vi "VI LogKonfig.vi"() -> ()   [LabVIEW 2020, in "LogKonfig.lvlib"]
uses:
  Seiten/Log Konfig/LogKonfig.lvlib
  Visualisierungs Elemente/String - Eingabefeld.ctl
  Visualisierungs Elemente/Pfad-Eingabefeld.ctl
  Visualisierungs Elemente/Button.ctl
  Visualisierungs Elemente/Auswahlfeld.ctl
  Visualisierungs Elemente/Zahlen-Eingabefeld.ctl
  Linearisierung V2/AktivButton.ctl
  Seiten/FT-IR/FGV FT-IR Aktionen.ctl
  Seiten/Log Konfig/Aktionen Logdatei erstellen.ctl
  Seiten/Log Konfig/Aktionen Trigger.ctl
  Seiten/FT-IR/FGV FT-IR Gasliste Aktionen.ctl
  Seiten/Log Konfig/Aktion LabBaseIndex.ctl
  Seiten/Log Konfig/Log Sequence FGV Aktion.ctl
  Passwortverwaltung/FGV Passwort Aktion.ctl
  SysLog/SysLog Interface.ctl
  Seiten/Log Konfig/Element Triggerereignisse.ctl
  Seiten/Log Konfig/Auswahlfeld aktiviert-deaktiviert.ctl
  Seiten/FT-IR/FT-IR.lvlib
  Seiten/FT-IR/TOOLweb Interface Library/TOOLweb Interface.lvlib
  Passwortverwaltung/Passwort.lvlib
  Allgemein/allgemeine Sub-VIs.lvlib
  Messdaten/Messdaten.lvlib
  SysLog/SysLog.lvlib
  Linearisierung V2/Linearisierung v2.lvlib
panel:
  in  "Registerkartenelement":T1(tab)
  out "Index Nr.":u32 caption="SPEC#:"
  in  "Index Nr. Start:":u32 caption="SPEC#:"
  in  "Logdatei erstellen":u16(ring) items=["Deaktiviert", "Aktiviert"]
  in  "Name":T2
  in  "Pfad LogDatei":T3
  in  "Trigger verwenden":u16(ring) items=["Deaktiviert", "Aktiviert"]
  in  "Puffergröße":T4 format="%#_5g"
  in  "Triggerereignis":T5
  in  "Messwert":T6 items=["---"]
  in  "kl./gr.":T6 items=["kleiner", "größer"]
  in  "Wert":T4 format="%#_5g"
  in  "Spektrum Loggen":u16(ring) items=["Deaktiviert", "Aktiviert"]
  in  "Pfad Spektren":T3
  in  "(82) labBaseName":T2
  in  "max. Größe  in Byte":u32=31457280 caption="max. Größe in Byte" min=15000 format="%#.0f"
  in  "Original Liste":i32(listbox)
  in  "Übernehmen":T5
  in  "Konfigurierte Liste":i32(listbox)
  in  "Löschen":T5
  in  "Alle Löschen":T5
  in  "Alle Übernehmen":T5
  in  "Spektrum File Name":T7 caption="Spektrum Datei Name"
  # "Log Konfig"
  # "FT-IR Spectrum"
  # "Spektrum Loggen?"
  # "Pfad für Spektren:"
  # "Bezeichnung:"
  # "Logdatei Messdaten"
  # "Logdatei erstellen?"
  # "Pfad für Logdatei:"
  # "Messreihenbezeichnung:"
  # "Trigger Einstellungen"
  # "-- Taste [F11]"
  # "--24V Trigger-Input"
  # "Trigger verwenden?"
  # "Triggerereignisse:"
  # "-- AK-Befehl [STRG]"
  # "sec"
  # "Puffergröße:"
  # "(Der Pufferbereich wird vor dem Triggerereignis mitgeloggt)"
  # "-- Messwert"
  # "Konfiguration Kanalreihenfolge"
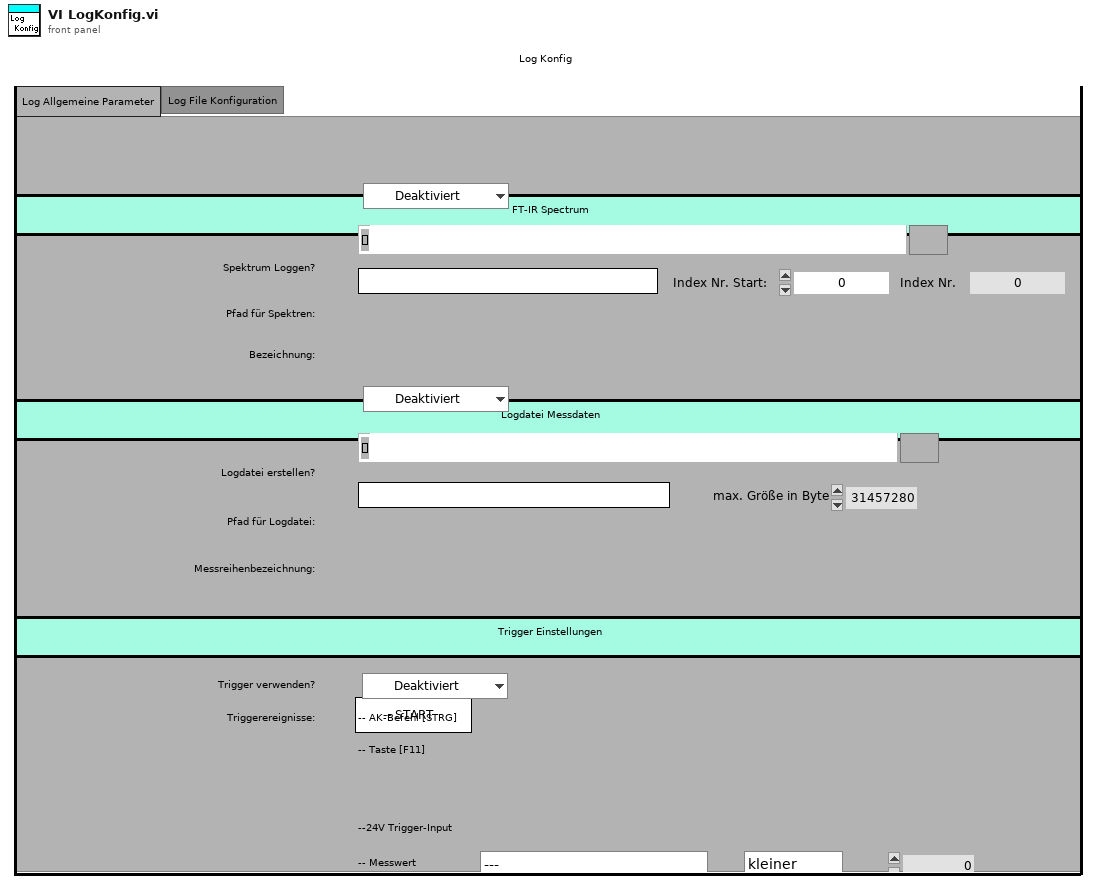
[diagram p1: front panel]
types:
  T1 = enum32{"Log General Parameter", "Log File Configuration"}
  T2 = typedef "String - Eingabefeld.ctl" = string
  T3 = typedef "Pfad-Eingabefeld.ctl" = path
  T4 = typedef "Zahlen-Eingabefeld.ctl" = sgl
  T5 = typedef "Button.ctl" = bool
  T6 = typedef "Auswahlfeld.ctl" = u16
  T7 = typedef "Linearisierung v2.lvlib/AktivButton.ctl" = bool
  T8 = typedef "LogKonfig.lvlib/Aktion LabBaseIndex.ctl" = enum16{"lesen", "schreiben"}
  T9 = typedef "FT-IR.lvlib/FGV FT-IR Gasliste Aktionen.ctl" = enum16{"lesen", "Gasliste FT-IR", "Gasliste ausgelesen", "laden", "speichern", "löschen"}
  T10 = typedef "LogKonfig.lvlib/Aktionen Trigger.ctl" = enum16{"lesen", "ALLE schreiben", "Trigger prüfen", "Trigger rücksetzen"}
  T11 = typedef "LogKonfig.lvlib/Aktionen Logdatei erstellen.ctl" = enum16{"lesen", "Logdatei erstellen NEU", "Name NEU", "Pfad NEU", "Log Stop", "max Size"}
  T12 = typedef "FT-IR.lvlib/FGV FT-IR Aktionen.ctl" = enum16{"lesen", "NOG setzen", "NOS setzen", "Initialisieren", "speichern", "ALLES setzen", "FT-IR Spektrum loggen", "Komm Stoppen", "Spektrum LogKonfig"}
  T13 = typedef "LogKonfig.lvlib/Log Sequence FGV Aktion.ctl" = enum16{"initialisieren", "lesen", "schreiben", "laden", "speichern", "übertragen"}
  T14 = typedef "LogKonfig.lvlib/Auswahlfeld aktiviert-deaktiviert.ctl" = u16
  T15 = typedef "LogKonfig.lvlib/Element Triggerereignisse.ctl" = cluster{"Trigger verwenden":T14, "Messwert":u16, "kl./gr.":u16, "Wert":sgl, "Puffergröße":sgl}
  T16 = cluster{"(80) labEnabled":bool, "(81) labPath":path, "(82) labBaseName":string, "(83) labIndex":string, "Spektrum loggen aktiv?":bool}
  T17 = typedef "String - Ausgabefeld.ctl" = string
  T18 = cluster{"Index Array":i32[], "Namen Array":string[], "Spektrum File Name":bool}
  T19 = typedef "Passwort.lvlib/FGV Passwort Aktion.ctl" = enum16{"prüfen", "setzen", "Initialisieren", "PW speichern", "lesen", "PW Änderung"}
  T20 = typedef "SysLog.lvlib/SysLog Interface.ctl" = cluster{"FehlermeldungsCode":i32, "ErfolgsmeldungsCode":i32, "ParameterListenString":string, "Anzeige":bool, "SysLogIcon":enum16{"OK", "Warnung", "Fehler"}, "intern":bool}
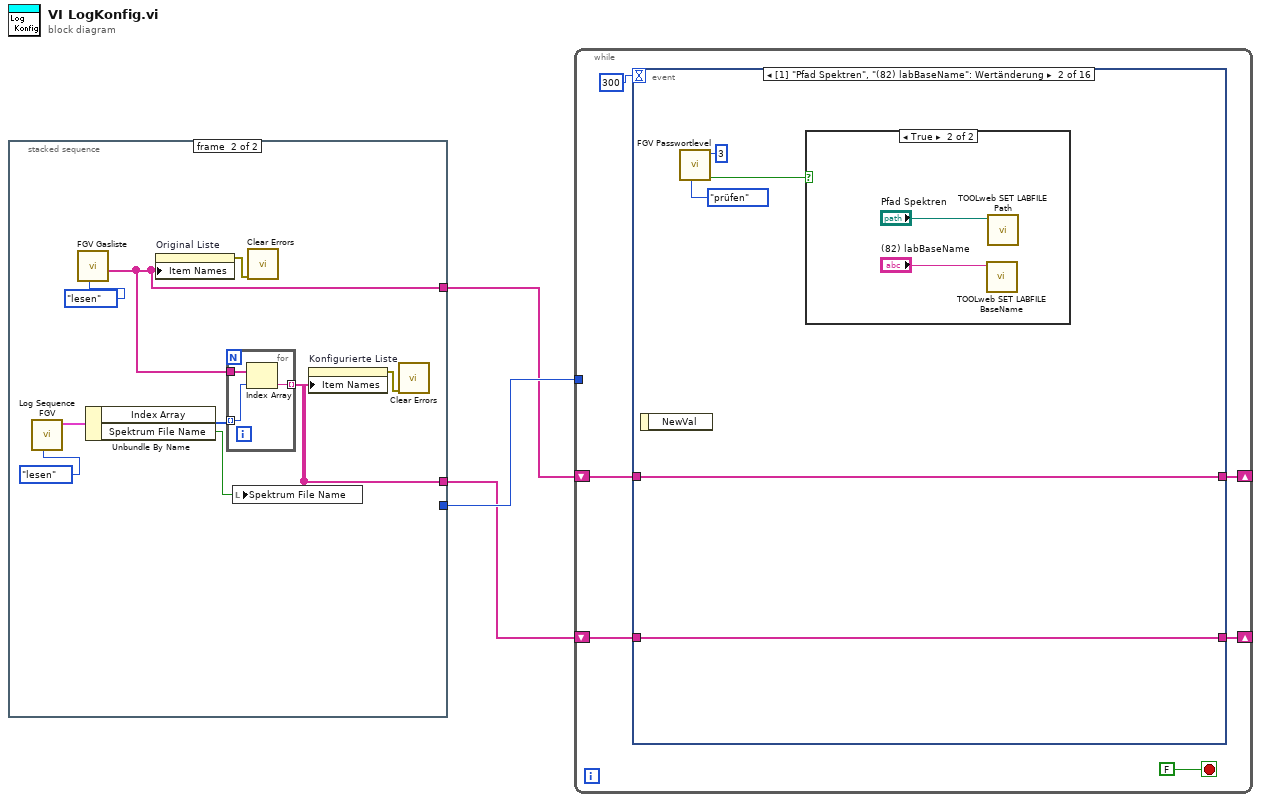
[diagram p0: block diagram]
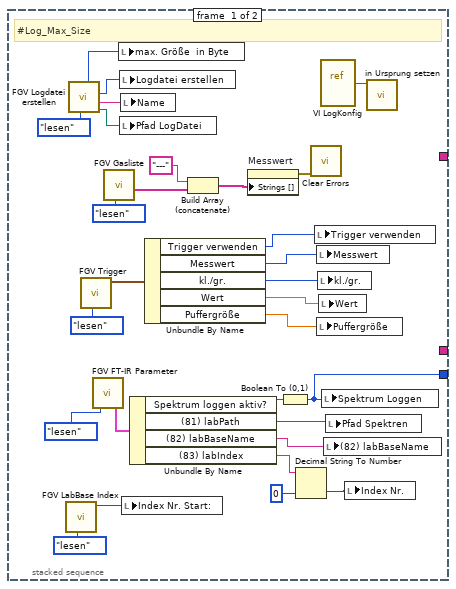
[diagram p2: hidden frame]
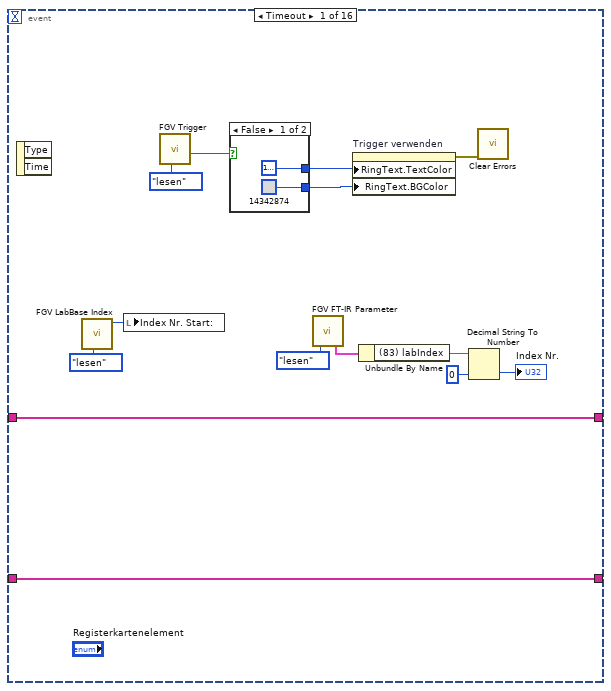
[diagram p3: hidden frame]
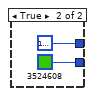
[diagram p4: hidden frame]
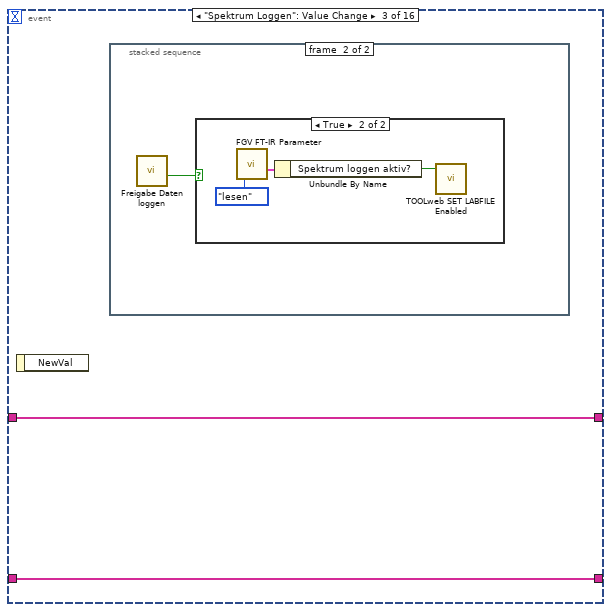
[diagram p6: hidden frame]
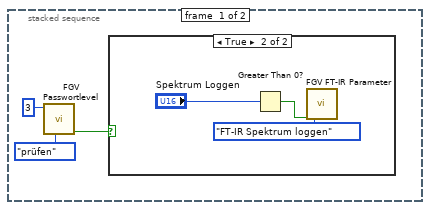
[diagram p7: hidden frame]
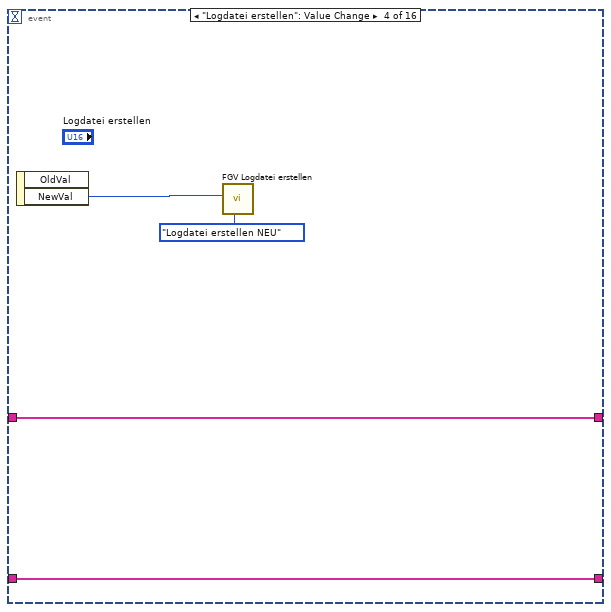
[diagram p10: hidden frame]
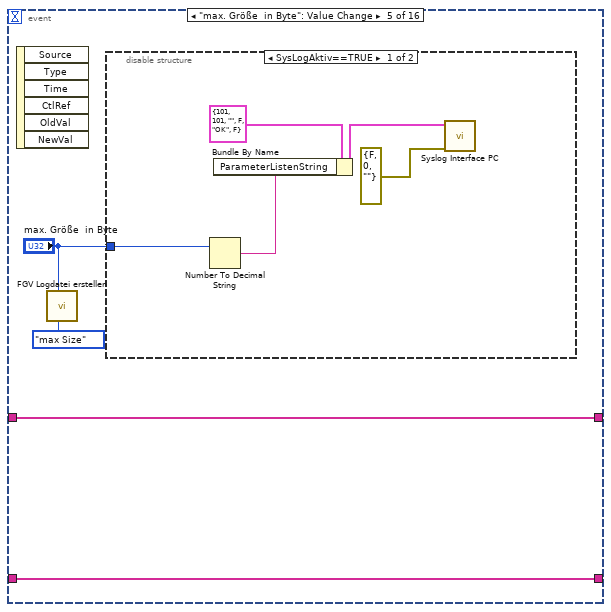
[diagram p11: hidden frame]
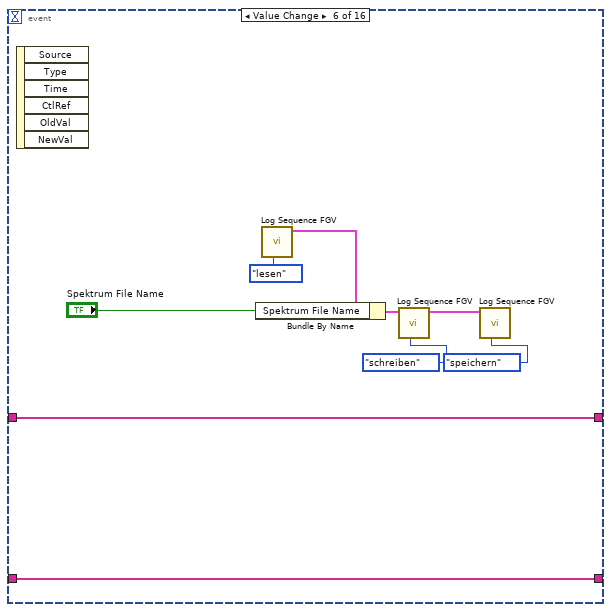
[diagram p13: hidden frame]
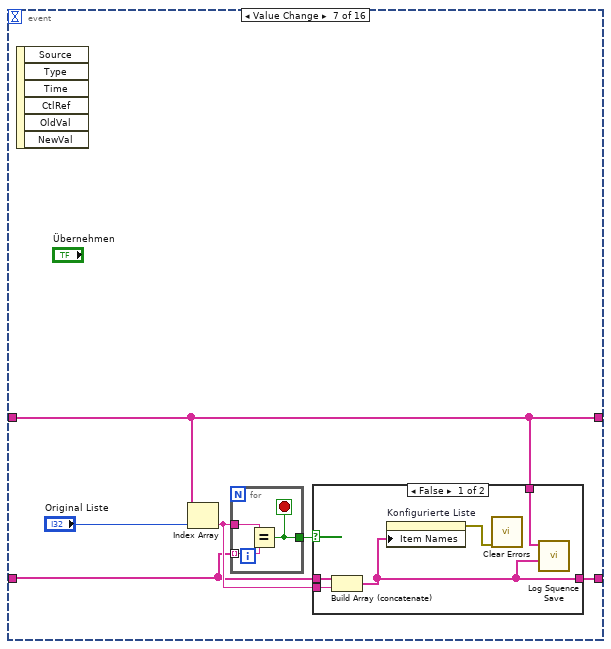
[diagram p14: hidden frame]
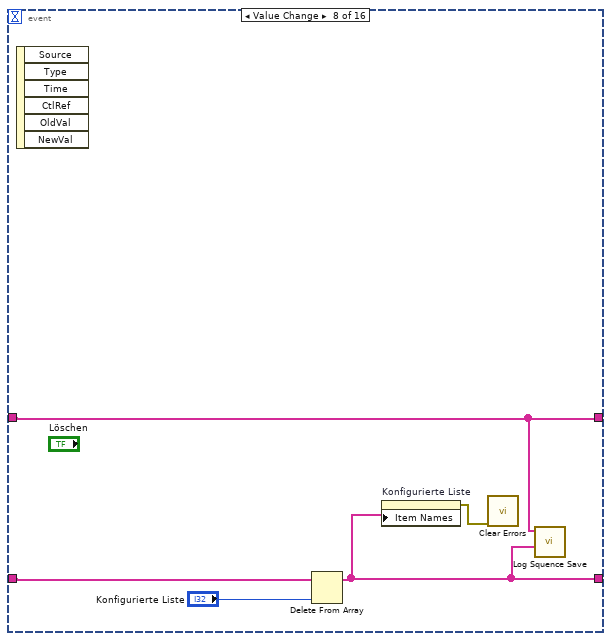
[diagram p16: hidden frame]
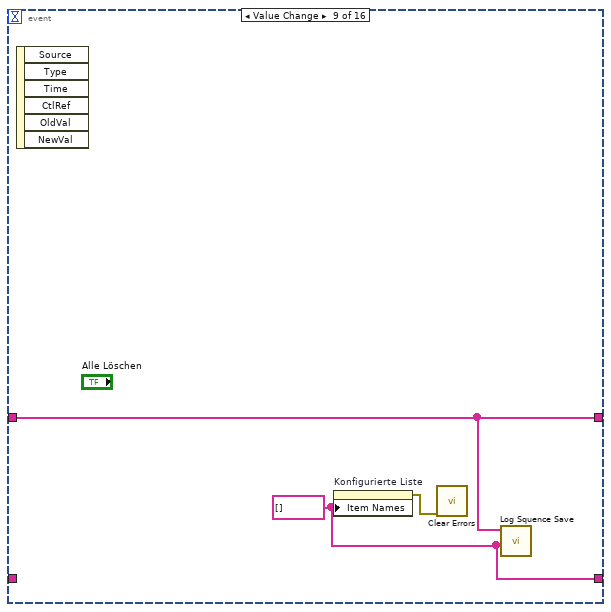
[diagram p17: hidden frame]
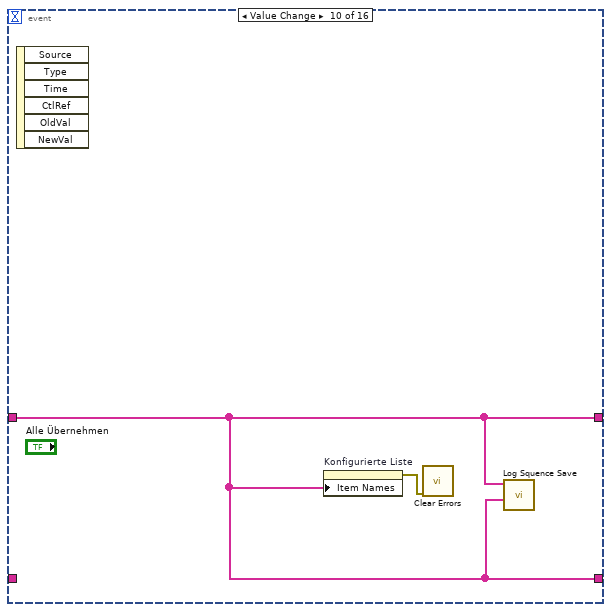
[diagram p18: hidden frame]
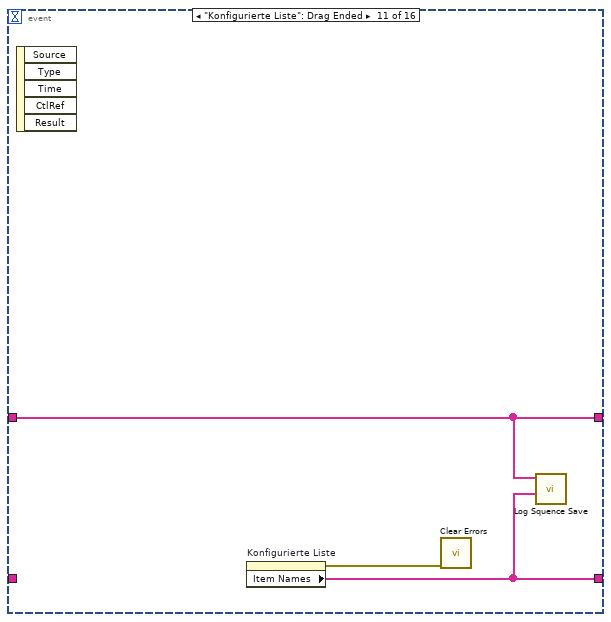
[diagram p19: hidden frame]
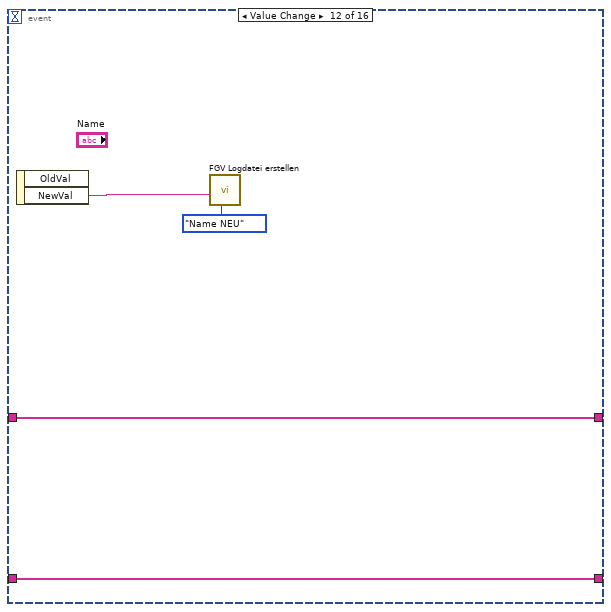
[diagram p20: hidden frame]
diagram:
  n1 = stacked-sequence {
    tunnel: [w17 _] -> w3
    tunnel: [_ w34] -> w1
    tunnel: [_ w33] -> w2
    frame #0 {
      # "#Log_Max_Size"
      n2 = call "FGV LabBase Index.vi"("Aktion"=Aktion_LabBaseIndex."lesen") -> ("Index Nr. Start:"=w7:u32)  [unwired: 9 in, 1 out]
      n3 = call "FGV Logdatei erstellen.vi"("Aktion"=Aktionen_Logdatei_erstellen."lesen") -> ("Pfad LogDatei neu"=w25:path, "Name Log Datei neu"=w26:string, "Logdatei erstellen neu"=w27:T14, "max. Größe  in Byte neu"=w9:i64)  [unwired: 6 in, 1 out]
      n4 = call "FGV Trigger.vi"("Aktion"=Aktionen_Trigger."lesen") -> ("Triggerereignis neu"=w19:T15)  [unwired: 7 in, 3 out]
      n5 = call "FGV FT-IR Parameter.vi"("Aktion"=FGV_FT-IR_Aktionen."lesen") -> ("Ausgangs-Cluster"=w31:T16)  [unwired: 11 in, 7 out]
      n6 = call "FGV Gasliste.vi"("Aktionen"=FGV_FT-IR_Gasliste_Aktionen."lesen") -> ("Aktuelle Gasliste gesamt"=w15:T17[])  [unwired: 8 in, 2 out]
      n7 = local write "max. Größe  in Byte"(w9) -> ()
      n8 = local write "Logdatei erstellen"(w27) -> ()
      n9 = local write "Pfad LogDatei"(w25) -> ()
      n10 = local write "Name"(w26) -> ()
      n11 = local write "Index Nr. Start:"(w7) -> ()
      n12 = Unbundle By Name(w31) -> ("Spektrum loggen aktiv?"=w18:bool, "(81) labPath"=w30:path, "(82) labBaseName"=w29:string, "(83) labIndex"=w4:string)
      n13 = Unbundle By Name(w19) -> ("Trigger verwenden"=w20:T14, "Messwert"=w12:u16, "kl./gr."=w23:u16, "Wert"=w22:sgl, "Puffergröße"=w21:sgl)
      n14 = Build Array (concatenate)("---" ("String"), w15) -> (w16:T17[])
      n15 = property on="Messwert" class="Ring (strikt)"("Strings []"=w16) -> (error out=w11:errorcluster)  [unwired: 2 in, 1 out]
      n16 = Boolean To (0,1)(Boolean=w18) -> (0, 1=w17:i16)
      n17 = Decimal String To Number(string=w4, default (0L)=u32 0 ("SPEC#:")) -> (number=w5:u32)  [unwired: 1 in, 1 out]
      n18 = call <vilib>:"Clear Errors.vi"("error in (no error)"=w11) -> ()  [unwired: 5 in, 2 out]
      n19 = local write "Trigger verwenden"(w20) -> ()
      n20 = local write "Messwert"(w12) -> ()
      n21 = local write "Puffergröße"(w21) -> ()
      n22 = local write "kl./gr."(w23) -> ()
      n23 = local write "Wert"(w22) -> ()
      n24 = vi-ref "VI LogKonfig.vi"() -> (w10:refnum<vi>)
      n25 = local write "Spektrum Loggen"(w17) -> ()
      n26 = local write "(82) labBaseName"(w29) -> ()
      n27 = local write "Pfad Spektren"(w30) -> ()
      n28 = local write "Index Nr."(w5) -> ()
      n29 = call "in Ursprung setzen.vi"("VI Referenz"=w10) -> ()  [unwired: 10 in, 1 out]
    }
    frame #1 {
      n30 = call "Log Sequence FGV.vi"("Aktion"=Log_Sequence_FGV_Aktion."lesen") -> ("Cluster (out)"=w38:T18)  [unwired: 10 in]
      n31 = call "FGV Gasliste.vi"("Aktionen"=FGV_FT-IR_Gasliste_Aktionen."lesen") -> ("Aktuelle Gasliste gesamt"=w33:T17[])  [unwired: 8 in, 2 out]
      n32 = Unbundle By Name(w38) -> ("Index Array"=w39:i32[], "Spektrum File Name"=w41:bool)
      n33 = property on="Original Liste" class="Listenfeld (strikt)"("Item Names"=w33) -> (error out=w37:errorcluster)  [unwired: 2 in, 1 out]
      n34 = for {
        tunnel: w39 -> [w44] mode=indexing
        tunnel: w33 -> [w43]
        tunnel: [w42] -> w34 mode=indexing
        n35 = Index Array(array=w43, index=w44) -> (element=w42:T17)
      }
      n36 = local write "Spektrum File Name"(w41) -> ()
      n37 = call <vilib>:"Clear Errors.vi"("error in (no error)"=w37) -> ()  [unwired: 5 in, 2 out]
      n38 = property on="Konfigurierte Liste" class="Listenfeld (strikt)"("Item Names"=w34) -> (error out=w40:errorcluster)  [unwired: 2 in, 1 out]
      n39 = call <vilib>:"Clear Errors.vi"("error in (no error)"=w40) -> ()  [unwired: 5 in, 2 out]
    }
  }
  n40 = while {
    tunnel: w3 -> [_]
    shift-right: [w45] -> _
    shift-left: w2 -> [w48]
    shift-right: [w46] -> _
    shift-left: w1 -> [w47]
    stop <- FALSE stop-if-true
    n41 = event shown="[1] \"Pfad Spektren\", \"(82) labBaseName\": Wertänderung" {
      selector: _ -> [_ _ _ _ _ _ _ _ _ _ _ _ _ _ _ _]
      dyn-events: _ -> [_ _ _ _ _ _ _ _ _ _ _ _ _ _ _ _]
      timeout: 300 -> [_ _ _ _ _ _ _ _ _ _ _ _ _ _ _ _]
      tunnel: w48 -> [w59 w70 w77 w89 w93 w108 w112 w126 w130 w133 w135 w139 w143 w147 w157 w168]
      tunnel: w47 -> [w58 w69 w76 w88 w92 w109 w111 w127 _ _ _ w138 w142 w146 w156 w169]
      tunnel: [w58 w69 w76 w88 w92 w109 w110 w125 w131 w133 w136 w138 w142 w146 w156 w169] -> w46
      tunnel: [w59 w70 w77 w89 w93 w108 w112 w126 w130 w133 w135 w139 w143 w147 w157 w168] -> w45
      event Timeout {
        n42 = event-data() -> ()  [unwired: 1 in, 2 out]
        n43 = call "FGV LabBase Index.vi"("Aktion"=Aktion_LabBaseIndex."lesen") -> ("Index Nr. Start:"=w57:u32)  [unwired: 9 in, 1 out]
        n44 = local write "Index Nr. Start:"(w57) -> ()
        n45 = call "FGV Trigger.vi"("Aktion"=Aktionen_Trigger."lesen") -> ("Trigger gesetzt?"=w64:bool)  [unwired: 7 in, 3 out]
        n46 = case shown="False" w64 {
          tunnel: [u32 16777222 u32 16777222] -> w61
          tunnel: [u32 14342874 u32 3524608] -> w62
          frame False {
          }
          frame True {
          }
        }
        n47 = call "FGV FT-IR Parameter.vi"("Aktion"=FGV_FT-IR_Aktionen."lesen") -> ("Ausgangs-Cluster"=w54:T16)  [unwired: 11 in, 7 out]
        n48 = property on="Trigger verwenden" class="Ring (strikt)"("RingText.TextColor"=w61, "RingText.BGColor"=w62) -> (error out=w60:errorcluster)  [unwired: 2 in, 1 out]
        n49 = Unbundle By Name(w54) -> ("(83) labIndex"=w52:string)
        n50 = Decimal String To Number(string=w52, default (0L)=u32 0 ("SPEC#:")) -> (number=→"Index Nr.":u32)  [unwired: 1 in, 1 out]
        n51 = call <vilib>:"Clear Errors.vi"("error in (no error)"=w60) -> ()  [unwired: 5 in, 2 out]
      }
      event Value Change {
        n52 = event-data() -> ()  [unwired: 1 in, 1 out]
        n53 = call "FGV Passwortlevel.vi"("FGV Passwort Aktion"=FGV_Passwort_Aktion."prüfen", "geforderter Level"=i16 3) -> ("Freigabe"=w73:bool)  [unwired: 2 in, 7 out]
        n54 = case shown="True" w73 {
          frame False {
          }
          frame True {
            n55 = call "TOOLweb SET LABFILE BaseName.vi"("BaseName"="(82) labBaseName") -> ()  [unwired: 2 in, 5 out]
            n56 = call "TOOLweb SET LABFILE Path.vi"("labPath"="Pfad Spektren") -> ()  [unwired: 2 in, 5 out]
          }
        }
      }
      event "Spektrum Loggen": Value Change {
        n57 = event-data() -> ()  [unwired: 1 in, 1 out]
        n58 = stacked-sequence {
          frame #0 {
            n59 = call "FGV Passwortlevel.vi"("FGV Passwort Aktion"=FGV_Passwort_Aktion."prüfen", "geforderter Level"=i16 3) -> ("Freigabe"=w78:bool)  [unwired: 2 in, 7 out]
            n60 = case shown="True" w78 {
              frame False {
              }
              frame True {
                n61 = Greater Than 0?(x="Spektrum Loggen") -> (x > 0?=w81:bool)
                n62 = call "FGV FT-IR Parameter.vi"("Spektrum loggen aktiv?"=w81, "Aktion"=FGV_FT-IR_Aktionen."FT-IR Spektrum loggen") -> ()  [unwired: 10 in, 8 out]
              }
            }
          }
          frame #1 {
            n63 = call "Freigabe Daten loggen.vi"() -> ("Daten loggen"=w84:bool)  [unwired: 11 in]
            n64 = case shown="True" w84 {
              frame False {
              }
              frame True {
                n65 = call "FGV FT-IR Parameter.vi"("Aktion"=FGV_FT-IR_Aktionen."lesen") -> ("Ausgangs-Cluster"=w87:T16)  [unwired: 11 in, 7 out]
                n66 = Unbundle By Name(w87) -> ("Spektrum loggen aktiv?"=w85:bool)
                n67 = call "TOOLweb SET LABFILE Enabled.vi"("Enabled"=w85) -> ()  [unwired: 2 in, 5 out]
              }
            }
          }
        }
      }
      event "Logdatei erstellen": Value Change {
        n68 = event-data() -> ("NewVal"=w91:u16)  [unwired: 1 in, 1 out]
        n69 = call "FGV Logdatei erstellen.vi"("Aktion"=Aktionen_Logdatei_erstellen."Logdatei erstellen NEU", "Logdatei erstellen"=w91) -> ()  [unwired: 5 in, 5 out]
      }
      event "max. Größe  in Byte": Value Change {
        n70 = event-data() -> ()  [unwired: 1 in, 6 out]
        n71 = call "FGV Logdatei erstellen.vi"("Aktion"=Aktionen_Logdatei_erstellen."max Size", "max. Größe  in Byte"="max. Größe  in Byte") -> ()  [unwired: 5 in, 5 out]
        n72 = disable-structure shown="SysLogAktiv==TRUE" {
          disable-tunnel: "max. Größe  in Byte" -> [w100 _]
          frame condition #0 (active) {
            n73 = Number To Decimal String(number=w100) -> (decimal integer string=w96:string)  [unwired: 1 in]
            n74 = Bundle By Name(cluster=T20 {"FehlermeldungsCode"=101, "ErfolgsmeldungsCode"=101, "ParameterListenString"="", "Anzeige"=FALSE, "SysLogIcon"=enum."OK", "intern"=FALSE} ("Cluster (in)"), "ParameterListenString"=w96) -> (w97:T20)
            n75 = call "Syslog Interface PC.vi"("Fehler (in)"=errorcluster {"status"=FALSE, "code"=0, "source"=""}, "Cluster (in)"=w97) -> ()  [unwired: 9 in, 1 out]
          }
          frame condition #1 {
          }
        }
      }
      event Value Change {
        n76 = event-data() -> ()  [unwired: 1 in, 6 out]
        n77 = call "Log Sequence FGV.vi"("Aktion"=Log_Sequence_FGV_Aktion."lesen") -> ("Cluster (out)"=w107:T18)  [unwired: 10 in]
        n78 = Bundle By Name(cluster=w107, "Spektrum File Name"="Spektrum File Name") -> (w105:T18)
        n79 = call "Log Sequence FGV.vi"("Aktion"=Log_Sequence_FGV_Aktion."schreiben", "Cluster (in)"=w105) -> ("Cluster (out)"=w106:T18)  [unwired: 9 in]
        n80 = call "Log Sequence FGV.vi"("Aktion"=Log_Sequence_FGV_Aktion."speichern", "Cluster (in)"=w106) -> ()  [unwired: 9 in, 1 out]
      }
      event Value Change {
        n81 = event-data() -> ()  [unwired: 1 in, 6 out]
        n82 = Index Array(array=w112, index="Original Liste") -> (element=w115:T17)
        n83 = for {
          tunnel: w115 -> [w124]
          tunnel: w111 -> [w123] mode=indexing
          tunnel: [w122] -> w114
          stop <- w122 stop-if-true
          n84 = Equal?(x=w124, y=w123) -> (x = y?=w122:bool)
        }
        n85 = case shown="False" w114 {
          tunnel: w111 -> [w119 w121]
          tunnel: [w117 w121] -> w110
          tunnel: w115 -> [w118 _]
          tunnel: w112 -> [w116 _]
          frame False {
            n86 = Build Array (concatenate)(w119, w118) -> (w117:T17[])
            n87 = property on="Konfigurierte Liste" class="Listenfeld (strikt)"("Item Names"=w117) -> (error out=w120:errorcluster)  [unwired: 2 in, 1 out]
            n88 = call <vilib>:"Clear Errors.vi"("error in (no error)"=w120) -> ()  [unwired: 5 in, 2 out]
            n89 = call "Log Squence Save.vi"("Item Names"=w117, "Aktuelle Gasliste gesamt"=w116) -> ()  [unwired: 9 in, 1 out]
          }
          frame True {
          }
        }
      }
      event Value Change {
        n90 = event-data() -> ()  [unwired: 1 in, 6 out]
        n91 = Delete From Array(array=w127, index="Konfigurierte Liste") -> (array with subset deleted=w125:T17[])  [unwired: 1 in, 1 out]
        n92 = property on="Konfigurierte Liste" class="Listenfeld (strikt)"("Item Names"=w125) -> (error out=w128:errorcluster)  [unwired: 2 in, 1 out]
        n93 = call <vilib>:"Clear Errors.vi"("error in (no error)"=w128) -> ()  [unwired: 5 in, 2 out]
        n94 = call "Log Squence Save.vi"("Item Names"=w125, "Aktuelle Gasliste gesamt"=w126) -> ()  [unwired: 9 in, 1 out]
      }
      event Value Change {
        w131 = string[] [] ("Objektnamen")
        n95 = event-data() -> ()  [unwired: 1 in, 6 out]
        n96 = property on="Konfigurierte Liste" class="Listenfeld (strikt)"("Item Names"=w131) -> (error out=w132:errorcluster)  [unwired: 2 in, 1 out]
        n97 = call <vilib>:"Clear Errors.vi"("error in (no error)"=w132) -> ()  [unwired: 5 in, 2 out]
        n98 = call "Log Squence Save.vi"("Item Names"=w131, "Aktuelle Gasliste gesamt"=w130) -> ()  [unwired: 9 in, 1 out]
      }
      event Value Change {
        n99 = event-data() -> ()  [unwired: 1 in, 6 out]
        n100 = property on="Konfigurierte Liste" class="Listenfeld (strikt)"("Item Names"=w133) -> (error out=w134:errorcluster)  [unwired: 2 in, 1 out]
        n101 = call <vilib>:"Clear Errors.vi"("error in (no error)"=w134) -> ()  [unwired: 5 in, 2 out]
        n102 = call "Log Squence Save.vi"("Item Names"=w133, "Aktuelle Gasliste gesamt"=w133) -> ()  [unwired: 9 in, 1 out]
      }
      event "Konfigurierte Liste": Drag Ended {
        n103 = event-data() -> ()  [unwired: 1 in, 5 out]
        n104 = property on="Konfigurierte Liste" class="Listenfeld (strikt)"() -> (error out=w137:errorcluster, "Item Names"=w136:string[])  [unwired: 2 in, 1 out]
        n105 = call <vilib>:"Clear Errors.vi"("error in (no error)"=w137) -> ()  [unwired: 5 in, 2 out]
        n106 = call "Log Squence Save.vi"("Item Names"=w136, "Aktuelle Gasliste gesamt"=w135) -> ()  [unwired: 9 in, 1 out]
      }
      event Value Change {
        n107 = event-data() -> ("NewVal"=w140:T2)  [unwired: 1 in, 1 out]
        n108 = call "FGV Logdatei erstellen.vi"("Aktion"=Aktionen_Logdatei_erstellen."Name NEU", "Name LogDatei"=w140) -> ()  [unwired: 5 in, 5 out]
      }
      event Value Change {
        # "#Log_Max_Size"
        n109 = event-data() -> ("NewVal"=w144:T3)  [unwired: 1 in, 1 out]
        n110 = call "FGV Logdatei erstellen.vi"("Aktion"=Aktionen_Logdatei_erstellen."Pfad NEU", "Pfad Log Datei"=w144) -> ()  [unwired: 5 in, 5 out]
      }
      event "Trigger verwenden": Value Change {
        n111 = event-data() -> ()  [unwired: 1 in, 1 out]
        n112 = Bundle By Name(cluster=T15 {"Trigger verwenden"=0, "Messwert"=0, "kl./gr."=0, "Wert"=0.0, "Puffergröße"=0.0} ("Triggerereignis"), "Trigger verwenden"="Trigger verwenden", "Messwert"="Messwert", "kl./gr."="kl./gr.", "Wert"="Wert", "Puffergröße"="Puffergröße") -> (w150:T15)
        n113 = call "FGV Trigger.vi"("Aktion"=Aktionen_Trigger."ALLE schreiben", "Triggerereignis"=w150) -> ()  [unwired: 6 in, 4 out]
      }
      event Value Change {
        n114 = event-data() -> ()  [unwired: 1 in, 1 out]
        n115 = call "FGV Trigger.vi"("Aktion"=Aktionen_Trigger."Trigger prüfen", "Trigger setzen"=TRUE) -> ()  [unwired: 6 in, 4 out]
      }
      event "Index Nr. Start:": Value Change {
        n116 = event-data() -> ()  [unwired: 1 in, 6 out]
        n117 = call "FGV FT-IR Parameter.vi"("Aktion"=FGV_FT-IR_Aktionen."lesen") -> ("Ausgangs-Cluster"=w161:T16)  [unwired: 11 in, 7 out]
        n118 = Number To Decimal String(number="Index Nr. Start:") -> (decimal integer string=w162:string)  [unwired: 1 in]
        n119 = call "TOOLweb SET LABINDEX.vi"("SPEC#:"="Index Nr. Start:") -> ("error out"=w164:errorcluster)  [unwired: 4 in, 2 out]
        n120 = Bundle By Name(cluster=w161, "(83) labIndex"=w162) -> (w160:T16)
        n121 = call "FGV LabBase Index.vi"("Aktion"=Aktion_LabBaseIndex."schreiben", "error in (no error)"=w164, "Index Nr. Start:"="Index Nr. Start:") -> ()  [unwired: 7 in, 2 out]
        n122 = call "FGV FT-IR Parameter.vi"("Ausgangs-Cluster"=w160, "Aktion"=FGV_FT-IR_Aktionen."Spektrum LogKonfig") -> ()  [unwired: 10 in, 8 out]
      }
    }
  }
